vi "Dashboard Main.vi"() -> ()   [LabVIEW 2013]
uses:
  <vilib>/event_ctls.llb/eventvkey.ctl
  <vilib>/Rock Robotics/WPI/Dashboard/WPI_DashboardLogging Global.vi
  <vilib>/Utility/config.llb/Write Key (String).vi
  <vilib>/Utility/config.llb/Write Key (I32).vi
  <vilib>/Utility/config.llb/NI_LVConfig.lvlib
panel:
  out "Image Message":string="Timeout in Camera Communications"
  in  "Rec Mode":enum32{"Stop", "Record", "Playback"}(radio)
  in  "Dashboard Tab":T1(tab)
  out "Auto-Grab Trigger":bool
  out "Arm Resting":bool
  out "Arm Pos":dbl
  in  "Retract Speed":dbl=0.4
  out "Motor2":dbl
  out "Motor1":dbl
  out "Launch":bool
  out "Grab":bool
  out "Launch Speed":dbl
  out "Launcher V":dbl
  in  "Pass Speed":dbl=-0.4
  in  "Max Launch Speed":dbl=-1.0
  in  "Pass V":dbl=2.8
  in  "Truss Launch V":dbl=1.7
  in  "Max Launch V":dbl=2.8
  in  "Camera Settings":T2={"Frame Rate"=30, "Compression"=30, "Size"=1} {"Frame Rate" scale=1.0..30.0; "Size" items=["640x480", "320x240", "160x120"]}
  out "MotorSliders R":cluster{"MotorSlide1":dbl, "MotorSlide2":dbl} {"MotorSlide2" scale=-1.0..1.0 scale format="%#_2e"; "MotorSlide1" scale=-1.0..1.0 scale format="%#_2e"}
  out "MotorChart R":cluster{"Numeric":dbl, "Numeric":dbl}(graph)
  out "MotorSliders L":T3 {"MotorSlide4 2" scale=0.0..14.0 scale format="%#_2e"; "MotorSlide2" scale=-1.0..1.0 scale format="%#_2e"; "MotorSlide1" scale=-1.0..1.0 scale format="%#_2e"}
  out "MotorChart L":T4(graph)
  out "JS1 Z":dbl(slide) scale=-1.0..1.0 scale format="%#_2e"
  out "Joystick 1":cluster{"X":dbl, "Y":dbl}[](graph)
  out "JS Buttons 1":T5
  out "JS2 Z":dbl(slide) scale=-1.0..1.0 scale format="%#_2e"
  out "Joystick 2":cluster{"X":dbl, "Y":dbl}[](graph)
  out "JS Buttons 2":T5
  out "Mode":T6(ring)=enum."Auto Disabled"
  out "Camera IP":string
  out "fps":dbl format="%#.1g"
  out "Mbps":dbl format="%#.1g"
  in  "DB Camera Config":bool
  in  "Enable":bool
  out "Mbps 2":bool
  in  "Horizontal":bool
  in  "Third":dbl=2000.0
  in  "Second":dbl=2500.0
  in  "Forward1":dbl=-0.8
  in  "First":dbl=2000.0
  in  "wait3":dbl=0.8
  in  "wait2":dbl
  in  "wait1":dbl
  in  "wait":dbl
  in  "Forward":dbl=-0.8 step=0.1
  in  "Test Slider":dbl(slide) scale=0.0..100.0 scale format="%#_3g"
  in  "On/Off":bool caption="Solenoid"
  in  "Test Name":u16(ring) items=["Select the test to run...", "Example Test", "-------------------------------", "List of tests is built in robot code.", "Replace with your own automated tests."]
  in  "Test Tree":string(tree)
  in  "Motor":cluster{"Value":dbl, "Enable":bool} {"Value" scale=-1.0..1.0 scale format="%#_3g"}
  out "Progress":T7 {"Test Progress" scale=0.0..100.0}
  in  "Rev/Fwd":cluster{"Forward":bool, "Reverse":bool}
  in  "Test Ring":u16(ring) items=["Auto", "Fixed indoor", "Fixed outdoor 1", "Fixed outdoor 2", "Fixed fluorescent 1", "Fixed fluorescent 2", "Hold current"]
  in  "Listbox":i32(listbox)
  out "Tree":string(tree)
  out "Camera Image":T8(plugin-control)
  # "Left"
  # "Front"
  # "Right"
  # "Battery"
  # "Customize by placing controls and indicators here and name to\nmatch Dashboard Variables on robot."
  # "This tab is a great place for autonomous settings and validation.\nCustomize by placing controls and indicators here and name to\nmatch Dashboard Variables on robot."
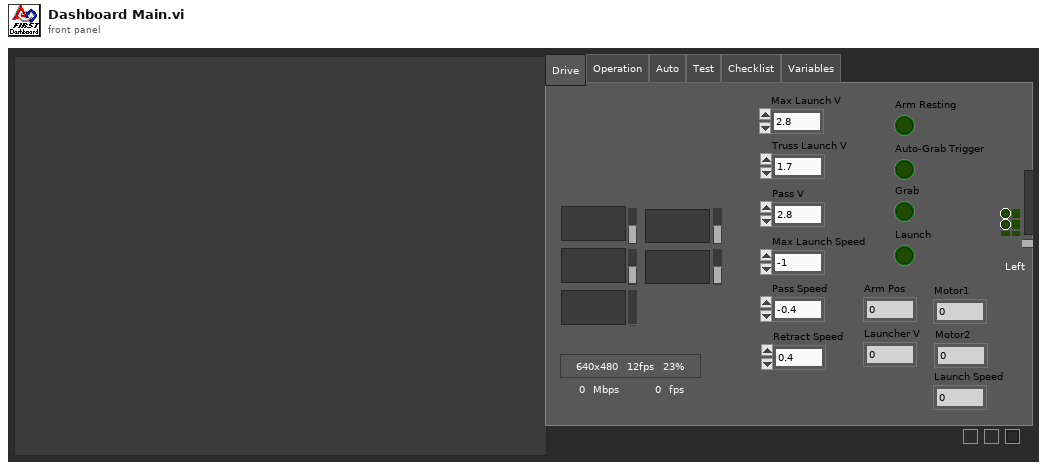
[diagram p1: front panel]
types:
  T1 = enum32{"Drive", "Operation", "Auto", "Test", "Checklist", "Variables"}
  T2 = cluster{"Frame Rate":i32, "Compression":i32, "Size":u16}
  T3 = cluster{"MotorSlide1":dbl, "MotorSlide2":dbl, "MotorSlide4 2":dbl}
  T4 = cluster{"Numeric":dbl, "Numeric":dbl, "Battery":sgl}
  T5 = cluster{bool, bool, bool, bool, bool, bool, bool, bool, bool, bool, bool, bool}
  T6 = enum8{"Tele-Op Disabled", "Tele-Op Enabled", "Auto Disabled", "Auto Enabled", "Test Disabled", "Test Enabled", ""}
  T7 = cluster{"Test Progress":u8, "Test Progress Text":string}
  T8 = typedef "IMAQ Image.ctl" = refnum<image>
  T9 = typedef "Image Type" = u32
  T10 = cluster{"Digital Inputs":bool[], "Digital Outputs":bool[]}
  T11 = cluster{"Competition mode":bool, "Robot Link":bool, "Autonomous":bool, "Enabled":bool, "E-Stop":bool, "Simulated":bool, "TestMode":bool, "Docked Window":bool}
  T12 = cluster{"wait":dbl, "wait1":dbl, "wait2":dbl, "wait3":dbl, "Forward":dbl, "Forward1":dbl, "First":dbl, "Second":dbl, "Third":dbl}
  T13 = cluster{"Boolean Array[0]":bool, "Boolean Array[1]":bool, "Boolean Array[2]":bool, "Boolean Array[3]":bool, "Boolean Array[4]":bool, "Boolean Array[5]":bool, "Boolean Array[6]":bool, "Boolean Array[7]":bool, "Boolean Array[8]":bool, "Boolean Array[9]":bool, "Boolean Array[10]":bool, "Boolean Array[11]":bool}
  T14 = typedef "NI_LVConfig.lvlib/Config Data RefNum.ctl" = refnum<k1>
  T15 = typedef "eventvkey.ctl" = enum16{"ASCII", "Enter", "Return", "Shift", "Ctrl", "Alt", "Cmd", "Opt", "Caps", "NumLock", "Clear", "Break", "Up", "Down", "Left", "Right", "Insert", "Delete", "Home", "End", "PageUp", "PageDown", "Escape", "Help", "Pause", "ScrollLock", "F1", "F2", "F3", "F4", "F5", "F6", "F7", "F8", "F9", "F10", "F11", "F12", "F13", "F14", "F15", "F16", "F17", "F18", "F19", "F20", "F21", "F22", "F23", "F24", "Play", "VolumeUp", "VolumeDown", "Mute", "Two Byte Char"}
  T16 = cluster{"Image Size":bool, "Image Type":bool, "Pixel Value":bool, "ROI Information":bool, "Zoom Factor":bool}
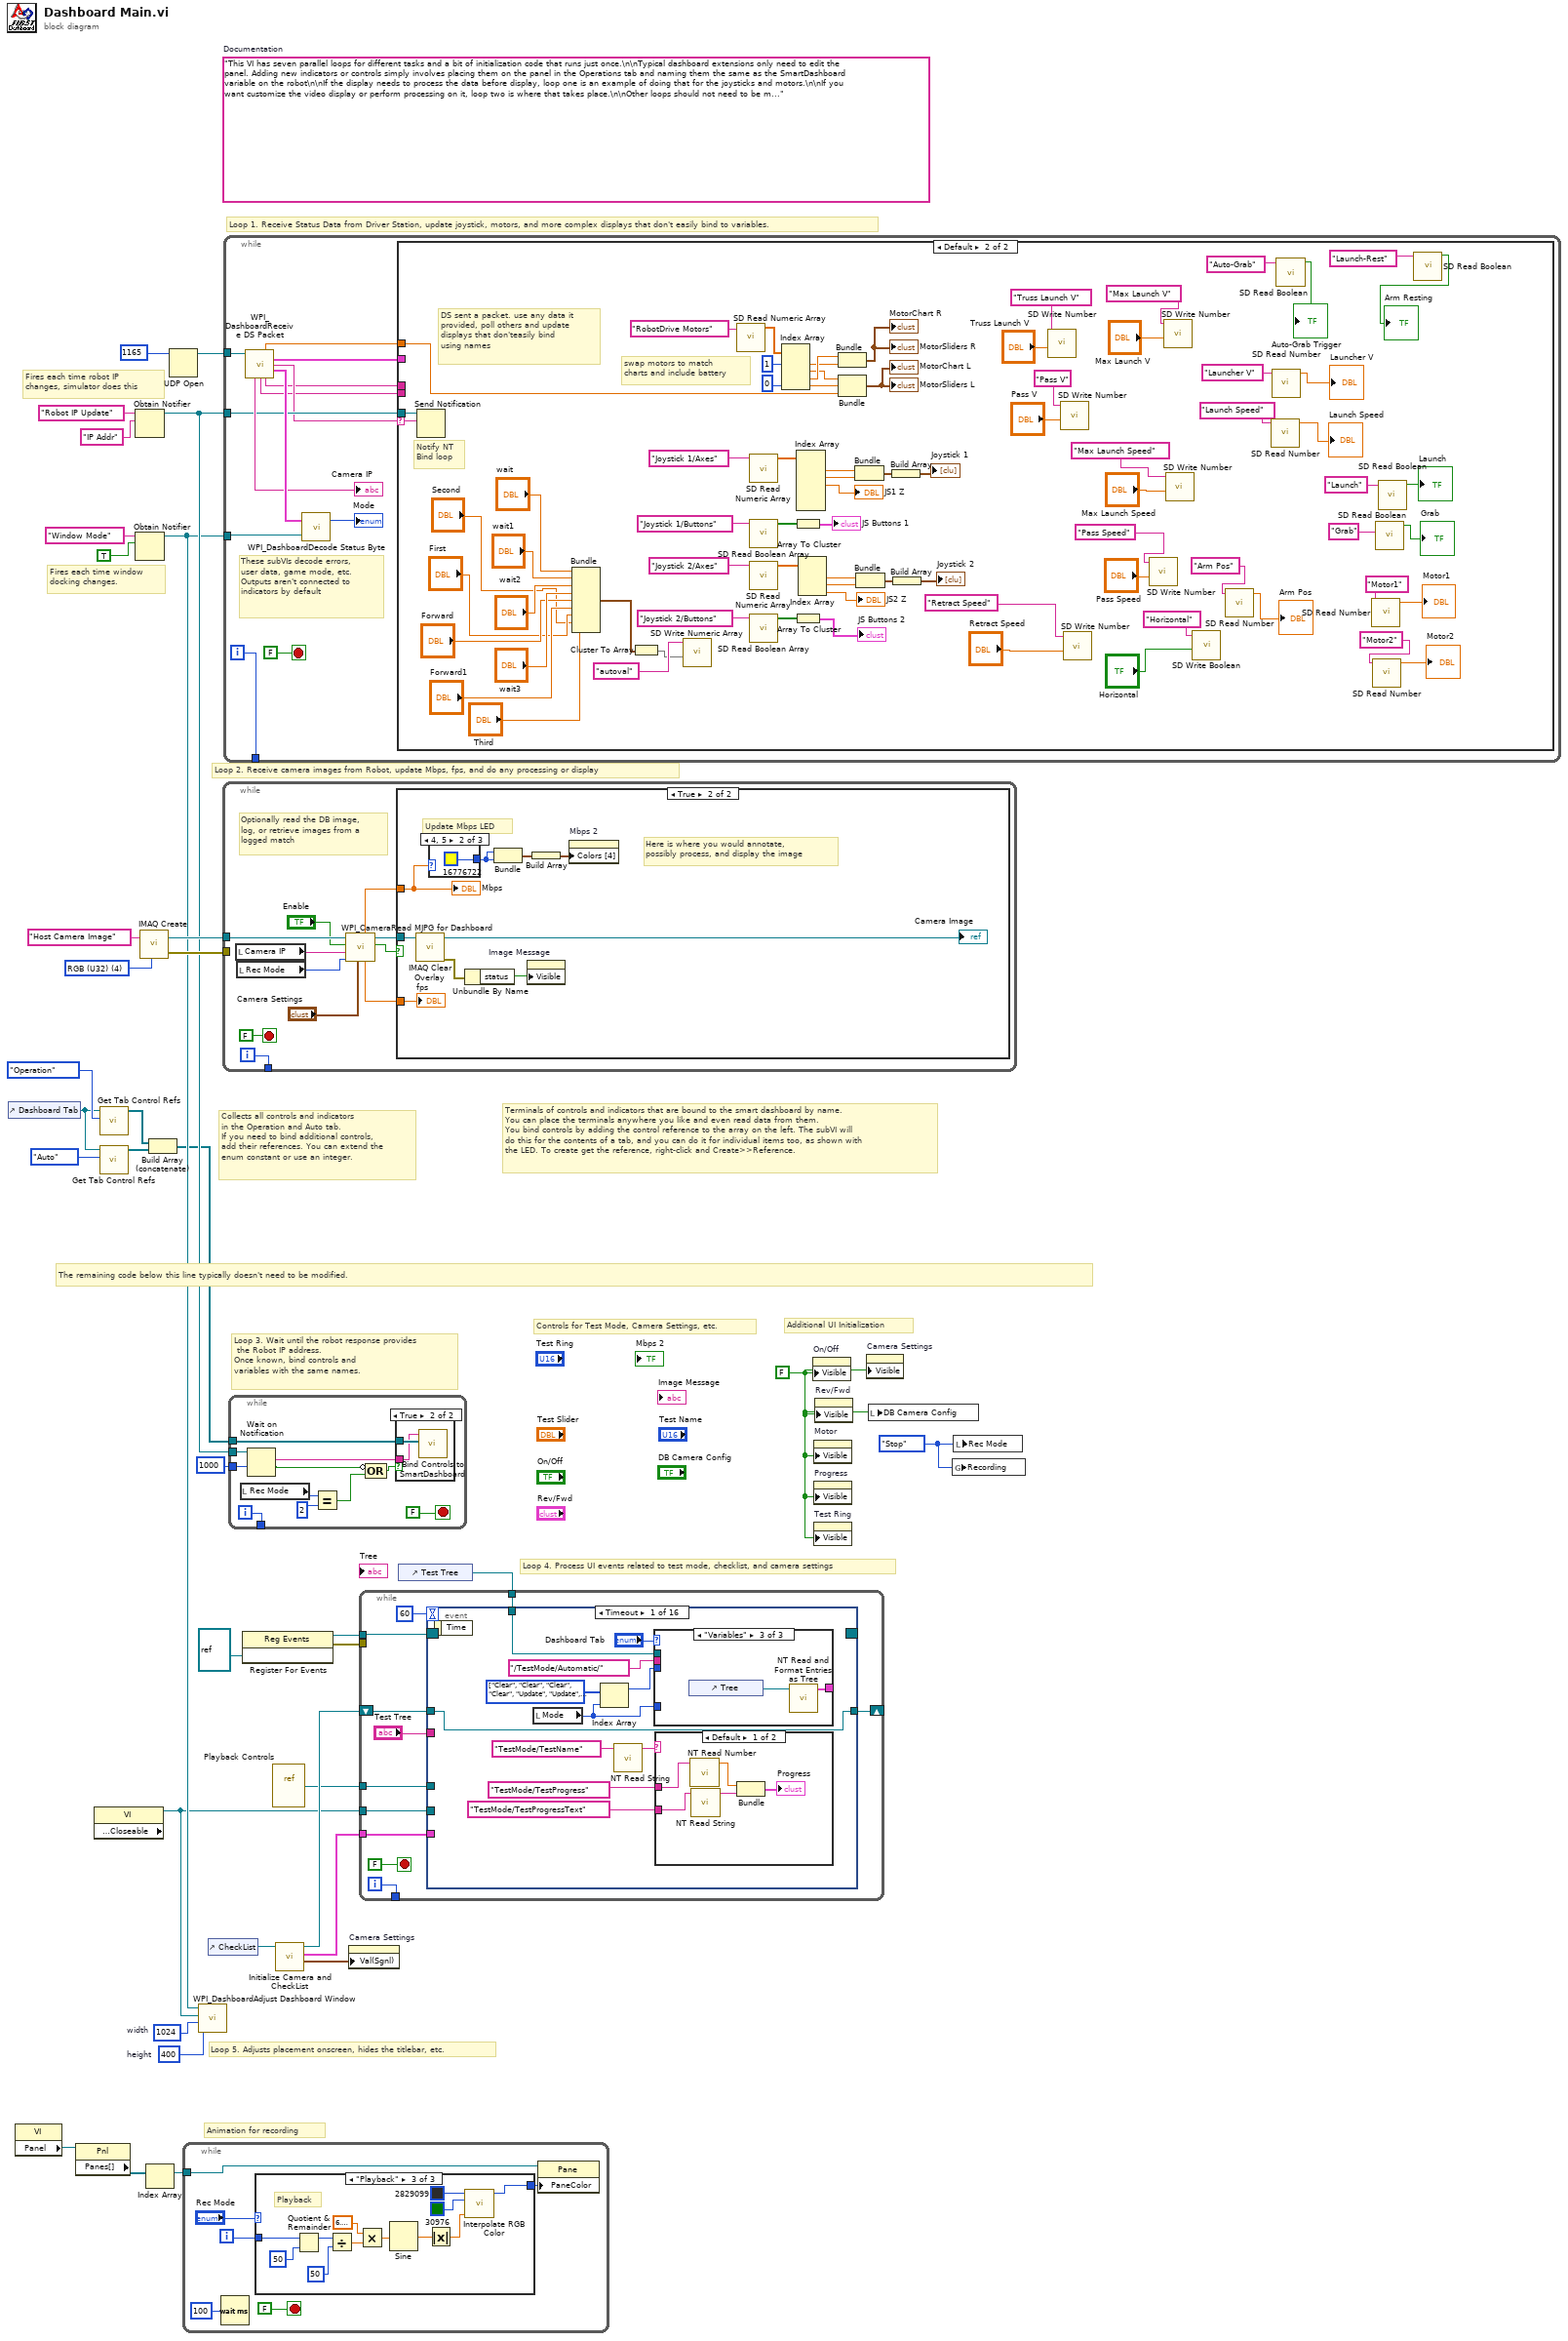
[diagram p0: block diagram]
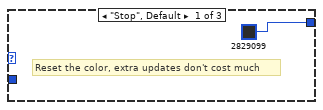
[diagram p2: hidden frame]
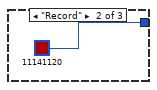
[diagram p3: hidden frame]
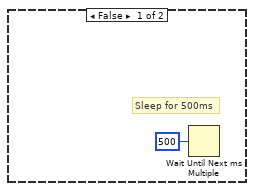
[diagram p5: hidden frame]
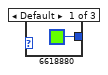
[diagram p6: hidden frame]
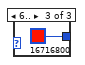
[diagram p7: hidden frame]
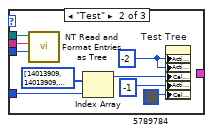
[diagram p9: hidden frame]
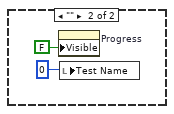
[diagram p10: hidden frame]
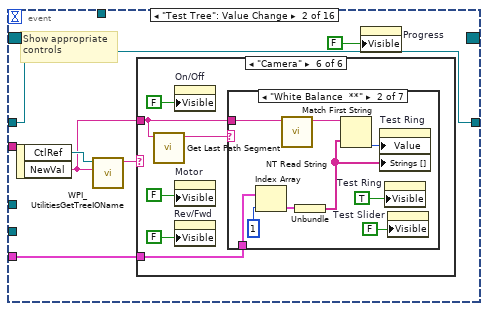
[diagram p11: hidden frame]
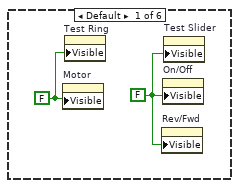
[diagram p12: hidden frame]
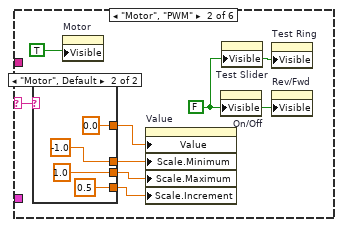
[diagram p13: hidden frame]
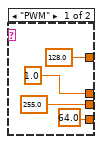
[diagram p14: hidden frame]
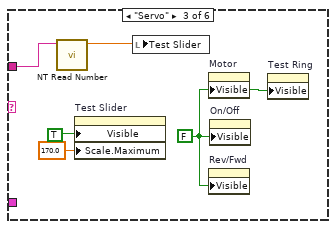
[diagram p15: hidden frame]
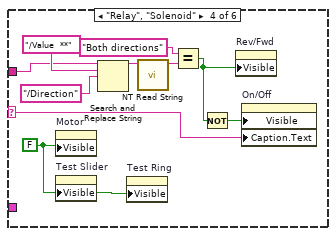
[diagram p16: hidden frame]
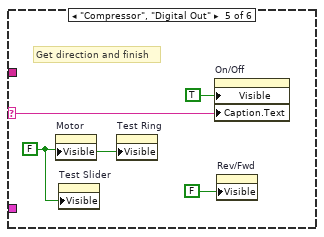
[diagram p17: hidden frame]
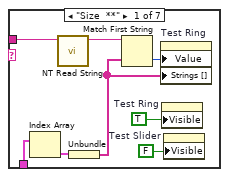
[diagram p18: hidden frame]
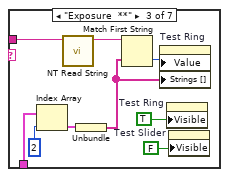
[diagram p19: hidden frame]
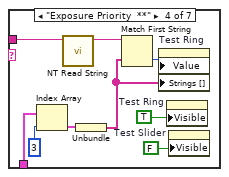
[diagram p20: hidden frame]
diagram:
  w7 = enum32{"Stop", "Record", "Playback"}."Stop" ("Rec Mode")
  w10 = 400  # height
  w11 = 1024  # width
  w24 = FALSE ("Visible")
  (unwired) "This VI has seven parallel loops for different tasks and a bit of initialization code that runs just once.\n\nTypical dashboard extensions only need to edit the panel. Adding new indicators or controls simply involves placing them on the panel in the Operations tab and naming them the same as the SmartDashboard variable on the robot\n\nIf the display needs to process the data before display, loop one is an example of doing that for the joysticks and motors.\n\nIf you want customize the video display or perform processing on it, loop two is where that takes place.\n\nOther loops should not need to be modified. They are pretty standard, and document the task they perform."  # Documentation
  w34 = T9 4 items=["Grayscale (U8)", "Grayscale (I16)", "Grayscale (SGL)", "Complex (CSG)", "RGB (U32)", "HSL (U32)", "RGB (U64)"] ("Image Type")
  # "Controls for Test Mode, Camera Settings, etc."
  # "Additional UI Initialization"
  # "Animation for recording"
  # "Fires each time robot IP\nchanges, simulator does this"
  # "Fires each time window\ndocking changes."
  # "Collects all controls and indicators\nin the Operation and Auto tab.\nIf you need to bind additional controls,\nadd their references. You can extend the\nenum constant or use an integer."
  # "The remaining code below this line typically doesn't need to be modified."
  # "Loop 4. Process UI events related to test mode, checklist, and camera settings"
  # "Terminals of controls and indicators that are bound to the smart dashboard by name.\nYou can place the terminals anywhere you like and even read data from them.\nYou bind controls by adding the control reference to the array on the left. The subVI will\ndo this for the contents of a tab, and you can do it for individual items too, as shown with\nthe LED. To create get the reference, right-click and Create>>Reference."
  # "Loop 3. Wait until the robot response provides\n the Robot IP address.\nOnce known, bind controls and\nvariables with the same names."
  # "Loop 5. Adjusts placement onscreen, hides the titlebar, etc."
  # "Loop 1. Receive Status Data from Driver Station, update joystick, motors, and more complex displays that don't easily bind to variables."
  # "Loop 2. Receive camera images from Robot, update Mbps, fps, and do any processing or display"
  n1 = control-ref of="Dashboard Tab"() -> (w5:refnum<vi>)
  n2 = property class="VI"() -> ("Panel"=w18:refnum<vi>)  [unwired: 2 in, 2 out]
  n3 = property class="Pnl"(reference=w18) -> ("Panes[]"=w19:refnum<vi>[])  [unwired: 1 in, 2 out]
  n4 = property class="VI" props=["Front Panel.Closeable"]() -> (reference out=w6:refnum<vi>)  [unwired: 2 in, 2 out]
  n5 = call <vilib>:"Get Tab Control Refs.vi"("Page Index"=T1."Operation" ("Dashboard Tab"), "TabControl in"=w5) -> ("ControlsOnPage"=w3:refnum<vi>[])  [unwired: 9 in]
  n6 = call <vilib>:"Get Tab Control Refs.vi"("Page Index"=T1."Auto" ("Dashboard Tab"), "TabControl in"=w5) -> ("ControlsOnPage"=w4:refnum<vi>[])  [unwired: 9 in]
  n7 = Obtain Notifier(name (unnamed)="Robot IP Update", notification data type="IP Addr" ("name (unnamed)")) -> (notifier out=w28:refnum<notifier>)  [unwired: 2 in, 2 out]
  n8 = Obtain Notifier(name (unnamed)="Window Mode", notification data type=TRUE) -> (notifier out=w9:refnum<notifier>)  [unwired: 2 in, 2 out]
  n9 = call "IMAQ Create"("Image Name"="Host Camera Image", "Image Type"=w34) -> ("New Image"=w32:T8, "error out"=w31:errorcluster)  [unwired: 2 in, 1 out]
  n10 = Index Array(array=w19) -> (element=w17:refnum<vi>)  [unwired: 1 in]
  n11 = Build Array (concatenate)(w3, w4) -> (w2:refnum<vi>[])
  n12 = UDP Open(11:u16 1165 ("port")) -> (port=w35:refnum<k16>)  [unwired: 2 in, 4 out]
  n13 = while {
    tunnel: w17 -> [w38]
    i -> [w41]
    stop <- FALSE stop-if-true
    n14 = Wait (ms)(milliseconds to wait=u32 100) -> ()  [unwired: 1 out]
    n15 = case shown="\"Playback\"" "Rec Mode" {
      tunnel: w41 -> [_ _ w56]
      tunnel: [u32 2829099 ("Base Color") u32 11141120 ("Target Color") w45] -> w37
      frame "Stop", Default {
        # "Reset the color, extra updates don't cost much"
      }
      frame "Record" {
      }
      frame "Playback" {
        # "Playback"
        n16 = Quotient & Remainder(x=w56, y=u32 50 ("milliseconds to wait")) -> (x-y*floor(x/y)=w52:u32)  [unwired: 1 out]
        n17 = Divide(x=w52, y=u32 50 ("milliseconds to wait")) -> (x/y=w49:dbl)
        n18 = Multiply(x=6.283185307179586, y=w49) -> (x*y=w54:dbl)
        n19 = Sine(x=w54) -> (sin(x)=w53:dbl)
        n20 = Absolute Value(x=w53) -> (abs(x)=w46:dbl)
        n21 = call "Interpolate RGB Color.vi"("Proportion"=w46, "Target Color"=u32 30976, "Base Color"=u32 2829099) -> ("Result Color"=w45:u32)  [unwired: 8 in]
      }
    }
    n22 = property class="Pane"(reference=w38, "PaneColor"=w37) -> ()  [unwired: 1 in, 2 out]
  }
  n23 = call <vilib>:"WPI_DashboardAdjust Dashboard Window.vi"("height"=w10, "width"=w11, "reference in"=w6, "Notifier in"=w9) -> ()  [unwired: 8 in]
  n24 = control-ref of="CheckList"() -> (w8:refnum<vi>)
  n25 = while {
    tunnel: w32 -> [w65]
    tunnel: w31 -> [_]
    tunnel: [w66] -> _
    i -> [w66]
    stop <- FALSE stop-if-true
    # "Optionally read the DB image,\nlog, or retrieve images from a\nlogged match"
    n26 = local read "Camera IP"() -> (w58:string)
    n27 = local read "Rec Mode"() -> (w57:enum32{"Stop", "Record", "Playback"})
    n28 = call <vilib>:"WPI_CameraRead MJPG for Dashboard.vi"("Camera Settings"="Camera Settings", "Rec Mode"=w57, "Camera IP"=w58, "Enable"="Enable", "Refnum in"=w65) -> ("Active"=w62:bool, "Refnum out"=w64:T8, "FPS"=w61:dbl, "Bandwidth (Mbps)"=w60:dbl)  [unwired: 3 in]
    n29 = case shown="True" w62 {
      tunnel: w64 -> [_ w72]
      tunnel: w60 -> [_ w71]
      tunnel: w61 -> [_ w69]
      frame False {
        # "Sleep for 500ms"
        n30 = Wait Until Next ms Multiple(millisecond multiple=u32 500) -> ()  [unwired: 1 out]
      }
      frame True {
        # "Here is where you would annotate,\npossibly process, and display the image"
        # "Update Mbps LED"
        n31 = call "IMAQ Clear Overlay"("Image"=w72) -> ("error out"=w76:errorcluster, "Image Out"=→"Camera Image":T8)  [unwired: 2 in, 7 out]
        n32 = case shown="4, 5" w71 {
          tunnel: [u32 6618880 ("Color Box") u32 16776722 ("Color Box") u32 16716800 ("Color Box")] -> w73
          frame Default {
          }
          frame 4, 5 {
          }
          frame 6.. {
          }
        }
        n33 = Unbundle By Name(w76) -> ("status"=w77:bool)
        n34 = Bundle("Color Box"=w73, "Color Box"=w73) -> (w75:cluster{"Color Box":u32, "Color Box":u32})  [unwired: 1 out]
        n35 = property on="Image Message" class="Str"("Visible"=w77) -> ()  [unwired: 2 in, 2 out]
        n36 = Build Array(w75) -> (w74:cluster{"Color Box":u32, "Color Box":u32}[])
        n37 = property on="Mbps 2" class="Bool (strict)"("Colors [4]"=w74) -> ()  [unwired: 2 in, 2 out]
        "Mbps" <- w71
        "fps" <- w69
      }
    }
  }
  n38 = while {
    tunnel: w35 -> [w91]
    tunnel: w28 -> [w86]
    tunnel: w9 -> [w90]
    tunnel: [w87] -> _
    i -> [w87]
    stop <- FALSE stop-if-true
    # "These subVIs decode errors, user data, game mode, etc.\nOutputs aren't connected to indicators by default"
    n39 = call <vilib>:"WPI_DashboardReceive DS Packet.vi"("Recv Socket"=w91) -> ("Battery"=w81:sgl, "Driver Station"=w82:T10, "Robot IP Address"=w85:string, "Status"=w92:T11, "Camera IP Address"=→"Camera IP":string, "Low Priority User Data"=w84:string, "High Priority User Data"=w83:string)  [unwired: 1 in, 7 out]
    n40 = call <vilib>:"WPI_DashboardDecode Status Byte.vi"("Window Mode Notifier"=w90, "Status"=w92) -> ("Mode"=→"Mode":T6)  [unwired: 1 out]
    n41 = case shown="Default" w85 {
      selector: w85 -> [_ w148]
      tunnel: w86 -> [_ w149]
      tunnel: w84 -> [_ _]
      tunnel: w83 -> [_ _]
      tunnel: w82 -> [_ _]
      tunnel: w81 -> [_ w147]
      frame "0.0.0.0" {
        # "DS not sending packets, or no robot exists yet.\nDon't poll the variables"
      }
      frame Default {
        # "Notify NT\nBind loop"
        # "DS sent a packet. use any data it\nprovided, poll others and update\ndisplays that don'teasily bind\nusing names"
        # "swap motors to match\ncharts and include battery"
        n42 = Send Notification(notification=w148, notifier=w149) -> ()  [unwired: 1 in, 2 out]
        n43 = Bundle("wait"="wait", "wait1"="wait1", "wait2"="wait2", "wait3"="wait3", "Forward"="Forward", "Forward1"="Forward1", "First"="First", "Second"="Second", "Third"="Third") -> (w103:T12)  [unwired: 1 in]
        n44 = Cluster To Array(cluster=w103) -> (array=w102:dbl[])
        n45 = call <vilib>:"SD Write Numeric Array.vi"("Numeric Array"=w102, "Name"="autoval") -> ()  [unwired: 8 in, 2 out]
        n46 = call <vilib>:"SD Read Numeric Array.vi"("Name"="RobotDrive Motors") -> ("Numeric Array"=w146:dbl[])  [unwired: 8 in, 2 out]
        n47 = call <vilib>:"SD Read Numeric Array.vi"("Name"="Joystick 1/Axes") -> ("Numeric Array"=w165:dbl[])  [unwired: 8 in, 2 out]
        n48 = call <vilib>:"SD Read Boolean Array.vi"("Name"="Joystick 1/Buttons") -> ("Boolean Array"=w167:bool[])  [unwired: 8 in, 2 out]
        n49 = call <vilib>:"SD Read Numeric Array.vi"("Name"="Joystick 2/Axes") -> ("Numeric Array"=w159:dbl[])  [unwired: 8 in, 2 out]
        n50 = call <vilib>:"SD Read Boolean Array.vi"("Name"="Joystick 2/Buttons") -> ("Boolean Array"=w158:bool[])  [unwired: 8 in, 2 out]
        n51 = Index Array(array=w146, index #1=1, index #4=0) -> (element #1=w142:dbl, element #2=w141:dbl, element #3=w143:dbl, element #4=w138:dbl)  [unwired: 2 in]
        n52 = Array To Cluster(array=w167) -> (cluster=→"JS Buttons 1":T13)
        n53 = Array To Cluster(array=w158) -> (cluster=→"JS Buttons 2":T13)
        n54 = Index Array(array=w165) -> (element #1=w162:dbl, element #2=w163:dbl, element #3=→"JS1 Z":dbl)  [unwired: 6 in, 3 out]
        n55 = Index Array(array=w159) -> (element #1=w154:dbl, element #2=w153:dbl, element #3=→"JS2 Z":dbl)  [unwired: 3 in]
        n56 = Bundle("Numeric"=w143, "Numeric"=w142) -> (→"MotorChart R" →"MotorSliders R":cluster{"Numeric":dbl, "Numeric":dbl})  [unwired: 1 in]
        n57 = Bundle("Numeric"=w141, "Numeric"=w138, "Battery"=w147) -> (→"MotorChart L" →"MotorSliders L":T4)  [unwired: 1 in]
        n58 = Bundle("Numeric"=w162, "Numeric"=w163) -> (w161:cluster{"Numeric":dbl, "Numeric":dbl})  [unwired: 1 in]
        n59 = Bundle("Numeric"=w154, "Numeric"=w153) -> (w155:cluster{"Numeric":dbl, "Numeric":dbl})  [unwired: 1 in]
        n60 = Build Array(w161) -> (→"Joystick 1":cluster{"Numeric":dbl, "Numeric":dbl}[])
        n61 = Build Array(w155) -> (→"Joystick 2":cluster{"Numeric":dbl, "Numeric":dbl}[])
        n62 = call <vilib>:"SD Write Number.vi"("Numeric"="Truss Launch V", "Name"="Truss Launch V") -> ()  [unwired: 8 in, 2 out]
        n63 = call <vilib>:"SD Write Number.vi"("Numeric"="Pass V", "Name"="Pass V") -> ()  [unwired: 8 in, 2 out]
        n64 = call <vilib>:"SD Write Number.vi"("Numeric"="Retract Speed", "Name"="Retract Speed") -> ()  [unwired: 8 in, 2 out]
        n65 = call <vilib>:"SD Write Number.vi"("Numeric"="Pass Speed", "Name"="Pass Speed") -> ()  [unwired: 8 in, 2 out]
        n66 = call <vilib>:"SD Write Number.vi"("Numeric"="Max Launch V", "Name"="Max Launch V") -> ()  [unwired: 8 in, 2 out]
        n67 = call <vilib>:"SD Write Number.vi"("Numeric"="Max Launch Speed", "Name"="Max Launch Speed") -> ()  [unwired: 8 in, 2 out]
        n68 = call <vilib>:"SD Write Boolean.vi"("Boolean"="Horizontal", "Name"="Horizontal") -> ()  [unwired: 8 in, 2 out]
        n69 = call <vilib>:"SD Read Number.vi"("Name"="Arm Pos") -> ("Numeric"=→"Arm Pos":dbl)  [unwired: 8 in, 2 out]
        n70 = call <vilib>:"SD Read Number.vi"("Name"="Launch Speed") -> ("Numeric"=→"Launch Speed":dbl)  [unwired: 8 in, 2 out]
        n71 = call <vilib>:"SD Read Number.vi"("Name"="Launcher V") -> ("Numeric"=→"Launcher V":dbl)  [unwired: 8 in, 2 out]
        n72 = call <vilib>:"SD Read Boolean.vi"("Name"="Auto-Grab") -> ("Boolean"=→"Auto-Grab Trigger":bool)  [unwired: 8 in, 2 out]
        n73 = call <vilib>:"SD Read Number.vi"("Name"="Motor1") -> ("Numeric"=→"Motor1":dbl)  [unwired: 8 in, 2 out]
        n74 = call <vilib>:"SD Read Number.vi"("Name"="Motor2") -> ("Numeric"=→"Motor2":dbl)  [unwired: 8 in, 2 out]
        n75 = call <vilib>:"SD Read Boolean.vi"("Name"="Grab") -> ("Boolean"=→"Grab":bool)  [unwired: 8 in, 2 out]
        n76 = call <vilib>:"SD Read Boolean.vi"("Name"="Launch") -> ("Boolean"=→"Launch":bool)  [unwired: 8 in, 2 out]
        n77 = call <vilib>:"SD Read Boolean.vi"("Name"="Launch-Rest") -> ("Boolean"=→"Arm Resting":bool)  [unwired: 8 in, 2 out]
      }
    }
  }
  n78 = while {
    tunnel: w2 -> [w181]
    tunnel: w28 -> [w179]
    tunnel: [w177] -> _
    tunnel: u32 1000 ("milliseconds to wait") -> [w176]
    i -> [w177]
    stop <- FALSE stop-if-true
    n79 = local read "Rec Mode"() -> (w172:enum32{"Stop", "Record", "Playback"})
    n80 = Wait on Notification(notifier=w179, timeout in ms (-1)=w176) -> (notification=w178:string, timed out?=w174:bool)  [unwired: 2 in, 2 out]
    n81 = Equal?(x=w172, y=u16 2 ("Rec Mode")) -> (x = y?=w173:bool)
    n82 = Compound Arithmetic op=OR(invert w174, w173) -> (w175:bool)
    n83 = case shown="True" w175 {
      tunnel: w181 -> [_ w183]
      tunnel: w178 -> [_ w182]
      frame False {
      }
      frame True {
        n84 = call <vilib>:"Bind Controls to SmartDashboard.vi"("Bound Control Refs"=w183, "Server IP Address"=w182) -> ()  [unwired: 10 in]
      }
    }
  }
  n85 = register-events(refnum<vi> refnum) -> (reference out=w15:refnum<event-registration>, error out=w14:errorcluster)  [unwired: 2 in]
  n86 = vi-ref "Playback Controls.vi"() -> (w16:refnum<vi>)
  n87 = call "Initialize Camera and CheckList.vi"("ListBox in"=w8) -> ("Cluster"=w22:cluster{"value":i32, "value":i32, "index":i32}, "Array"=w23:cluster{string[]}[], "File Refnum"=w21:T14)  [unwired: 8 in]
  n88 = property on="Camera Settings" class="Clust (strict)"("Val(Sgnl)"=w22) -> ()  [unwired: 2 in, 2 out]
  n89 = control-ref of="Test Tree"() -> (w20:refnum<vi>)
  n90 = while {
    tunnel: w23 -> [w191]
    shift-right: [w190] -> _
    shift-left: w21 -> [w189]
    tunnel: [w188] -> _
    tunnel: w20 -> [w187]
    tunnel: w16 -> [w186]
    tunnel: w15 -> [w185]
    tunnel: w14 -> [_]
    tunnel: w6 -> [w184]
    i -> [w188]
    stop <- FALSE stop-if-true
    n91 = event shown="[0] Timeout" {
      selector: w185 -> [_ _ _ _ _ _ _ _ _ _ _ _ _ _ _ _]
      dyn-events: [_ _ _ _ _ _ _ _ _ _ _ _ _ w429 _ _] -> _
      timeout: u32 60 ("milliseconds to wait") -> [_ _ _ _ _ _ _ _ _ _ _ _ _ _ _ _]
      tunnel: w187 -> [w201 _ _ _ _ _ _ _ _ _ _ _ _ _ _ _]
      tunnel: "Test Tree" -> [_ _ _ _ _ _ _ _ w398 w406 w408 w412 w420 _ _ _]
      tunnel: w191 -> [_ w225 _ _ _ _ w362 w392 _ _ _ _ _ _ _ _]
      tunnel: [w195 w224 w323 w328 w336 w348 w361 w385 w397 w404 w407 w411 w419 w431 w445 w446] -> w190
      tunnel: w189 -> [w195 w224 w323 w328 w336 w348 w360 w385 w397 w404 w407 w411 w419 w431 w445 w446]
      tunnel: w186 -> [_ _ _ _ _ _ _ _ _ _ _ _ _ w432 _ w449]
      tunnel: w184 -> [_ _ _ _ _ _ _ _ _ _ _ _ _ w427 _ _]
      event Timeout {
        w200 = enum16{"Update", "Clear"}[] [enum."Clear", enum."Clear", enum."Clear", enum."Clear", enum."Update", enum."Update", enum."Clear"] items=["Update", "Clear"]
        n92 = event-data() -> ()  [unwired: 1 in, 1 out]
        n93 = local read "Mode"() -> (w198:T6)
        n94 = Index Array(array=w200, index=w198) -> (element=w199:enum16{"Update", "Clear"})
        n95 = call <vilib>:"NT Read String.vi"("Name"="TestMode/TestName") -> ("String"=w204:string)  [unwired: 9 in, 1 out]
        n96 = case shown="\"Variables\"" "Dashboard Tab" {
          tunnel: w201 -> [_ w214 _]
          tunnel: "/TestMode/Automatic/" ("Name Pattern") -> [_ w213 _]
          tunnel: w199 -> [_ w212 _]
          tunnel: w198 -> [_ w210 _]
          tunnel: [_ _ w216] -> _
          frame "Operation", Default {
          }
          frame "Test" {
            w209 = -2 ("Active Item:Row Number")
            n97 = call <vilib>:"NT Read and Format Entries as Tree.vi"("Operation"=w212, "Name Pattern"=w213, "Tree Refnum"=w214) -> ()  [unwired: 7 in, 2 out]
            n98 = Index Array(array=u32[] [14013909, 14013909, 14013909, 14013909, 14013909, 16777215, 14013909], index=w210) -> (element=w208:u32)
            n99 = property on="Test Tree" class="Tree (strict)"("Active Item Row Number"=w209, "ActiveColNum"=w209, "CellBG"=w208, "Active Item Row Number"=-1 ("Active Item:Row Number"), "CellBG"=u32 5789784 ("Color Box")) -> ()  [unwired: 2 in, 2 out]
          }
          frame "Variables" {
            n100 = control-ref of="Tree"() -> (w215:refnum<vi>)
            n101 = call <vilib>:"NT Read and Format Entries as Tree.vi"("Tree Refnum"=w215) -> ("Formatted Strings"=w216:cluster{"Name":string, "Value":string}[])  [unwired: 9 in, 1 out]
          }
        }
        n102 = case shown="Default" w204 {
          tunnel: "TestMode/TestProgress" ("Name") -> [w218 _]
          tunnel: "TestMode/TestProgressText" ("Name") -> [w217 _]
          frame Default {
            n103 = call <vilib>:"NT Read Number.vi"("Name"=w218) -> ("Numeric"=w219:dbl)  [unwired: 9 in, 1 out]
            n104 = call <vilib>:"NT Read String.vi"("Name"=w217) -> ("String"=w220:string)  [unwired: 9 in, 1 out]
            n105 = Bundle("Numeric"=w219, "String"=w220) -> (→"Progress":cluster{"Numeric":dbl, "String":string})  [unwired: 1 in]
          }
          frame "" {
            n106 = property on="Progress" class="Clust (strict)"("Visible"=FALSE) -> ()  [unwired: 2 in, 2 out]
            n107 = local write "Test Name"(u16 0) -> ()
          }
        }
      }
      event "Test Tree": Value Change {
        # "Show appropriate\ncontrols"
        n108 = event-data() -> ("CtlRef"=w228:refnum<vi>, "NewVal"=w226:string)  [unwired: 1 in]
        n109 = call <vilib>:"WPI_UtilitiesGetTreeIOName.vi"("NewVal"=w226, "TreeControl in"=w228) -> ("I/O Name"=w229:string)  [unwired: 9 in]
        n110 = case shown="\"Camera\"" w229 {
          selector: w229 -> [_ w236 _ w254 w263 _]
          tunnel: w226 -> [_ _ w251 w253 _ w270]
          tunnel: w225 -> [_ _ _ _ _ w269]
          frame Default {
            w231 = FALSE ("Visible")
            w230 = FALSE ("Visible")
            n111 = property on="Motor" class="Clust (strict)"("Visible"=w230) -> ()  [unwired: 2 in, 2 out]
            n112 = property on="Test Ring" class="Ring (strict)"("Visible"=w230) -> ()  [unwired: 2 in, 2 out]
            n113 = property on="Rev/Fwd" class="Clust (strict)"("Visible"=w231) -> ()  [unwired: 2 in, 2 out]
            n114 = property on="On/Off" class="Bool (strict)"("Visible"=w231) -> ()  [unwired: 2 in, 2 out]
            n115 = property on="Test Slider" class="Slide (strict)"("Visible"=w231) -> ()  [unwired: 2 in, 2 out]
          }
          frame "Motor", "PWM" {
            w237 = FALSE ("Visible")
            n116 = case shown="\"Motor\", Default" w236 {
              tunnel: [1.0 ("Value") -1.0 ("Value")] -> w235
              tunnel: [255.0 ("Value") 1.0 ("Value")] -> w234
              tunnel: [128.0 ("Value") 0.0 ("Value")] -> w233
              tunnel: [64.0 ("Value") 0.5 ("Value")] -> w232
              frame "PWM" {
              }
              frame "Motor", Default {
              }
            }
            n117 = property on="Motor" class="Clust (strict)"("Visible"=TRUE) -> ()  [unwired: 2 in, 2 out]
            n118 = property on="Value" class="Slide (strict)"("Value"=w233, "Scale.Minimum"=w235, "Scale.Maximum"=w234, "Scale.Increment"=w232) -> ()  [unwired: 2 in, 2 out]
            n119 = property on="On/Off" class="Bool (strict)"("Visible"=w237) -> ()  [unwired: 2 in, 2 out]
            n120 = property on="Test Slider" class="Slide (strict)"("Visible"=w237) -> ()  [unwired: 2 in, 2 out]
            n121 = property on="Test Ring" class="Ring (strict)"("Visible"=w237) -> ()  [unwired: 2 in, 2 out]
            n122 = property on="Rev/Fwd" class="Clust (strict)"("Visible"=w237) -> ()  [unwired: 2 in, 2 out]
          }
          frame "Servo" {
            w249 = FALSE ("Visible")
            n123 = call <vilib>:"NT Read Number.vi"("Name"=w251) -> ("Numeric"=w250:dbl)  [unwired: 9 in, 1 out]
            n124 = property on="Test Slider" class="Slide (strict)"("Visible"=TRUE, "Scale.Maximum"=170.0 ("Scale.Range:Maximum")) -> ()  [unwired: 2 in, 2 out]
            n125 = local write "Test Slider"(w250) -> ()
            n126 = property on="Motor" class="Clust (strict)"("Visible"=w249) -> ()  [unwired: 2 in, 2 out]
            n127 = property on="Rev/Fwd" class="Clust (strict)"("Visible"=w249) -> ()  [unwired: 2 in, 2 out]
            n128 = property on="On/Off" class="Bool (strict)"("Visible"=w249) -> ()  [unwired: 2 in, 2 out]
            n129 = property on="Test Ring" class="Ring (strict)"("Visible"=w249) -> ()  [unwired: 2 in, 2 out]
          }
          frame "Relay", "Solenoid" {
            w252 = FALSE ("Visible")
            n130 = property on="Motor" class="Clust (strict)"("Visible"=w252) -> ()  [unwired: 2 in, 2 out]
            n131 = property on="Test Slider" class="Slide (strict)"("Visible"=w252) -> ()  [unwired: 2 in, 2 out]
            n132 = Search and Replace String(input string=w253, search string="/Value  **", replace string="/Direction") -> (result string=w259:string)  [unwired: 5 in, 3 out]
            n133 = property on="Test Ring" class="Ring (strict)"("Visible"=w252) -> ()  [unwired: 2 in, 2 out]
            n134 = call <vilib>:"NT Read String.vi"("Name"=w259) -> ("String"=w257:string)  [unwired: 9 in, 1 out]
            n135 = Equal?(x="Both directions", y=w257) -> (x = y?=w255:bool)
            n136 = Not(x=w255) -> (.not. x?=w256:bool)
            n137 = property on="Rev/Fwd" class="Clust (strict)"("Visible"=w255) -> ()  [unwired: 2 in, 2 out]
            n138 = property on="On/Off" class="Bool (strict)"("Visible"=w256, "Caption.Text"=w254) -> ()  [unwired: 2 in, 2 out]
          }
          frame "Compressor", "Digital Out" {
            w262 = FALSE ("Visible")
            # "Get direction and finish"
            n139 = property on="Motor" class="Clust (strict)"("Visible"=w262) -> ()  [unwired: 2 in, 2 out]
            n140 = property on="Test Slider" class="Slide (strict)"("Visible"=w262) -> ()  [unwired: 2 in, 2 out]
            n141 = property on="Test Ring" class="Ring (strict)"("Visible"=w262) -> ()  [unwired: 2 in, 2 out]
            n142 = property on="On/Off" class="Bool (strict)"("Visible"=TRUE, "Caption.Text"=w263) -> ()  [unwired: 2 in, 2 out]
            n143 = property on="Rev/Fwd" class="Clust (strict)"("Visible"=FALSE) -> ()  [unwired: 2 in, 2 out]
          }
          frame "Camera" {
            n144 = call <vilib>:"Get Last Path Segment.vi"("String in"=w270) -> ("String out"=w271:string)  [unwired: 10 in]
            n145 = property on="On/Off" class="Bool (strict)"("Visible"=FALSE) -> ()  [unwired: 2 in, 2 out]
            n146 = property on="Motor" class="Clust (strict)"("Visible"=FALSE) -> ()  [unwired: 2 in, 2 out]
            n147 = property on="Rev/Fwd" class="Clust (strict)"("Visible"=FALSE) -> ()  [unwired: 2 in, 2 out]
            n148 = case shown="\"White Balance  **\"" w271 {
              tunnel: w270 -> [w277 w286 w295 w304 w313 _ w319]
              tunnel: w269 -> [w275 w283 w292 w301 w310 _ _]
              frame "Size  **" {
                n149 = Index Array(array=w275) -> (element=w274:cluster{string[]})  [unwired: 1 in]
                n150 = call <vilib>:"NT Read String.vi"("Name"=w277) -> ("String"=w276:string)  [unwired: 9 in, 1 out]
                n151 = Unbundle(w274) -> (w272:string[])
                n152 = Match First String(2:w272, 3:w276) -> (0:w273:i32)  [unwired: 1 out]
                n153 = property on="Test Ring" class="Ring (strict)"("Value"=w273, "Strings []"=w272) -> ()  [unwired: 2 in, 2 out]
                n154 = property on="Test Ring" class="Ring (strict)"("Visible"=TRUE) -> ()  [unwired: 2 in, 2 out]
                n155 = property on="Test Slider" class="Slide (strict)"("Visible"=FALSE) -> ()  [unwired: 2 in, 2 out]
              }
              frame "White Balance  **" {
                n156 = Index Array(array=w283, index=1) -> (element=w284:cluster{string[]})
                n157 = call <vilib>:"NT Read String.vi"("Name"=w286) -> ("String"=w285:string)  [unwired: 9 in, 1 out]
                n158 = Unbundle(w284) -> (w281:string[])
                n159 = Match First String(2:w281, 3:w285) -> (0:w280:i32)  [unwired: 1 out]
                n160 = property on="Test Ring" class="Ring (strict)"("Value"=w280, "Strings []"=w281) -> ()  [unwired: 2 in, 2 out]
                n161 = property on="Test Ring" class="Ring (strict)"("Visible"=TRUE) -> ()  [unwired: 2 in, 2 out]
                n162 = property on="Test Slider" class="Slide (strict)"("Visible"=FALSE) -> ()  [unwired: 2 in, 2 out]
              }
              frame "Exposure  **" {
                n163 = Index Array(array=w292, index=2) -> (element=w293:cluster{string[]})
                n164 = call <vilib>:"NT Read String.vi"("Name"=w295) -> ("String"=w294:string)  [unwired: 9 in, 1 out]
                n165 = Unbundle(w293) -> (w289:string[])
                n166 = Match First String(2:w289, 3:w294) -> (0:w290:i32)  [unwired: 1 out]
                n167 = property on="Test Ring" class="Ring (strict)"("Value"=w290, "Strings []"=w289) -> ()  [unwired: 2 in, 2 out]
                n168 = property on="Test Ring" class="Ring (strict)"("Visible"=TRUE) -> ()  [unwired: 2 in, 2 out]
                n169 = property on="Test Slider" class="Slide (strict)"("Visible"=FALSE) -> ()  [unwired: 2 in, 2 out]
              }
              frame "Exposure Priority  **" {
                n170 = Index Array(array=w301, index=3) -> (element=w302:cluster{string[]})
                n171 = call <vilib>:"NT Read String.vi"("Name"=w304) -> ("String"=w303:string)  [unwired: 9 in, 1 out]
                n172 = Unbundle(w302) -> (w298:string[])
                n173 = Match First String(2:w298, 3:w303) -> (0:w299:i32)  [unwired: 1 out]
                n174 = property on="Test Ring" class="Ring (strict)"("Value"=w299, "Strings []"=w298) -> ()  [unwired: 2 in, 2 out]
                n175 = property on="Test Ring" class="Ring (strict)"("Visible"=TRUE) -> ()  [unwired: 2 in, 2 out]
                n176 = property on="Test Slider" class="Slide (strict)"("Visible"=FALSE) -> ()  [unwired: 2 in, 2 out]
              }
              frame "Color Enable  **" {
                n177 = Index Array(array=w310, index=4) -> (element=w311:cluster{string[]})
                n178 = call <vilib>:"NT Read String.vi"("Name"=w313) -> ("String"=w312:string)  [unwired: 9 in, 1 out]
                n179 = Unbundle(w311) -> (w307:string[])
                n180 = Match First String(2:w307, 3:w312) -> (0:w308:i32)  [unwired: 1 out]
                n181 = property on="Test Ring" class="Ring (strict)"("Value"=w308, "Strings []"=w307) -> ()  [unwired: 2 in, 2 out]
                n182 = property on="Test Ring" class="Ring (strict)"("Visible"=TRUE) -> ()  [unwired: 2 in, 2 out]
                n183 = property on="Test Slider" class="Slide (strict)"("Visible"=FALSE) -> ()  [unwired: 2 in, 2 out]
              }
              frame Default {
                n184 = property on="Test Ring" class="Ring (strict)"("Visible"=FALSE) -> ()  [unwired: 2 in, 2 out]
                n185 = property on="Test Slider" class="Slide (strict)"("Visible"=FALSE) -> ()  [unwired: 2 in, 2 out]
              }
              frame "Brightness  **", "Color Level  **", "Compression  **", "FPS  **", "Sharpness  **" {
                n186 = call <vilib>:"NT Read Number.vi"("Name"=w319) -> ("Numeric"=w318:dbl)  [unwired: 9 in, 1 out]
                n187 = local write "Test Slider"(w318) -> ()
                n188 = property on="Test Slider" class="Slide (strict)"("Visible"=TRUE, "Scale.Maximum"=100.0 ("Scale.Range:Maximum")) -> ()  [unwired: 2 in, 2 out]
                n189 = property on="Test Ring" class="Ring (strict)"("Visible"=FALSE) -> ()  [unwired: 2 in, 2 out]
              }
            }
          }
        }
        n190 = property on="Progress" class="Clust (strict)"("Visible"=FALSE) -> ()  [unwired: 2 in, 2 out]
      }
      event "Test Name": Mouse Enter {
        # "Populate the ring with the list of tests"
        n191 = event-data() -> ()  [unwired: 1 in, 1 out]
        n192 = call <vilib>:"NT Read String Array.vi"("Name"="TestMode/TestList") -> ("String Array"=w327:string[])  [unwired: 9 in, 1 out]
        n193 = Build Array (concatenate)("Select the test to run...", w327) -> (w326:string[])
        n194 = property on="Test Name" class="Ring (strict)"("Strings []"=w326) -> ()  [unwired: 2 in, 2 out]
      }
      event "Test Name": Value Change {
        w329 = FALSE ("Visible")
        # "Tell the robot the test name to run"
        n195 = event-data() -> ("NewVal"=w333:u16)  [unwired: 1 in]
        n196 = property on="Test Name" class="Ring (strict)"() -> ("Strings []"=w334:string[])  [unwired: 2 in, 2 out]
        n197 = local write "Progress"(T7 {"Test Progress"=0, "Test Progress Text"=""} ("Progress")) -> ()
        n198 = Index Array(array=w334, index=w333) -> (element=w332:string)
        n199 = call <vilib>:"NT Write String.vi"("String"=w332, "Name"="TestMode/TestName") -> ()  [unwired: 9 in, 1 out]
        n200 = property on="Progress" class="Clust (strict)"("Visible"=TRUE) -> ()  [unwired: 2 in, 2 out]
        n201 = property on="Motor" class="Clust (strict)"("Visible"=w329) -> ()  [unwired: 2 in, 2 out]
        n202 = property on="Test Slider" class="Slide (strict)"("Visible"=w329) -> ()  [unwired: 2 in, 2 out]
        n203 = property on="On/Off" class="Bool (strict)"("Visible"=w329) -> ()  [unwired: 2 in, 2 out]
        n204 = property on="Rev/Fwd" class="Clust (strict)"("Visible"=w329) -> ()  [unwired: 2 in, 2 out]
        n205 = property on="Test Ring" class="Ring (strict)"("Visible"=w329) -> ()  [unwired: 2 in, 2 out]
      }
      event "Listbox": Double Click {
        n206 = event-data() -> ("PlatMods.Shift"=w337:bool, "Row"=w339:i32)  [unwired: 1 in]
        n207 = case shown="True" w337 {
          tunnel: w339 -> [w343 _]
          tunnel: 1 -> [w342 _]
          frame False {
            n208 = property on="Listbox" class="LstBox (strict)"() -> ("Item Symbols"=w341:i32[])  [unwired: 2 in, 2 out]
            n209 = Replace Array Subset(array=w341, new element=w342, index=w343) -> (w340:i32[])
            n210 = property on="Listbox" class="LstBox (strict)"("Item Symbols"=w340) -> ()  [unwired: 2 in, 2 out]
          }
          frame True {
            w344 = 0 ("Top Row")
            n211 = property on="Listbox" class="LstBox (strict)"() -> ("Number of Rows"=w346:u32)  [unwired: 2 in, 2 out]
            n212 = Initialize Array(0, w346) -> (w345:i32[])
            n213 = property on="Listbox" class="LstBox (strict)"("Top Row"=w344, "Value"=w344, "Item Symbols"=w345) -> ()  [unwired: 2 in, 2 out]
          }
        }
      }
      event "Listbox": Key Down {
        n214 = event-data() -> ("VKey"=w350:T15)  [unwired: 1 in]
        n215 = case shown="\"Left\", \"Right\"" w350 {
          selector: w350 -> [w355 _]
          tunnel: eventvkey."Left" ("VKey") -> [w353 _]
          frame "Left", "Right" {
            n216 = Equal?(x=w353, y=w355) -> (x = y?=w354:bool)
            n217 = Select(t=0, s=w354, f=1) -> (s? t:f=w356:i32)
            n218 = property on="Listbox" class="LstBox (strict)"() -> ("Item Symbols"=w359:i32[])  [unwired: 2 in, 2 out]
            n219 = Replace Array Subset(array=w359, new element=w356, index="Listbox") -> (w358:i32[])
            n220 = property on="Listbox" class="LstBox (strict)"("Item Symbols"=w358) -> ()  [unwired: 2 in, 2 out]
          }
          frame Default {
          }
        }
      }
      event "DB Camera Config": Value Change {
        n221 = event-data() -> ("NewVal"=w363:bool)  [unwired: 1 in]
        n222 = case shown="False" w363 {
          tunnel: w362 -> [w372 _]
          tunnel: [w365 w383] -> w361
          tunnel: w360 -> [w364 w383]
          frame False {
            w379 = "Camera"
            w382 = FALSE ("Visible")
            n223 = local read "Camera Settings"() -> (w371:T2)
            n224 = Index Array(array=w372) -> (element=w375:cluster{string[]})  [unwired: 1 in]
            n225 = Unbundle(w371) -> ("Frame Rate"=w370:i32, "Compression"=w369:i32, "Size"=w373:u16)
            n226 = Unbundle(w375) -> (w374:string[])
            n227 = Index Array(array=w374, index=w373) -> (element=w368:string)
            n228 = call-poly <vilib>:"Write Key.vi"("section"=w379, "value"=w368, "key"="Size", "refnum"=w364) -> ("refnum out"=w381:T14)  [unwired: 2 in, 5 out]
            n229 = call-poly <vilib>:"Write Key.vi"("section"=w379, "value"=w370, "key"="FrameRate", "refnum"=w381) -> ("refnum out"=w380:T14)  [unwired: 1 in, 6 out]
            n230 = property on="Camera Settings" class="Clust (strict)"("Visible"=w382) -> ()  [unwired: 2 in, 2 out]
            n231 = local write "DB Camera Config"(w382) -> ()
            n232 = call-poly <vilib>:"Write Key.vi"("section"=w379, "value"=w369, "key"="Compression", "refnum"=w380) -> ("refnum out"=w366:T14)  [unwired: 1 in, 6 out]
            n233 = call <vilib>:"Close Config Data.vi"("refnum"=w366) -> ("file path"=w367:path)  [unwired: 2 in, 8 out]
            n234 = call <vilib>:"Open Config Data.vi"("configuration file path"=w367) -> ("refnum"=w365:T14)  [unwired: 8 in, 2 out]
          }
          frame True {
            n235 = property on="Camera Settings" class="Clust (strict)"("Visible"=TRUE) -> ()  [unwired: 2 in, 2 out]
          }
        }
      }
      event "Camera Settings": Value Change {
        n236 = event-data() -> ("NewVal"=w396:T2)  [unwired: 1 in]
        n237 = Index Array(array=w392) -> (element=w391:cluster{string[]})  [unwired: 1 in]
        n238 = Unbundle(w396) -> ("Frame Rate"=w387:i32, "Compression"=w386:i32, "Size"=w389:u16)
        n239 = Unbundle(w391) -> (w390:string[])
        n240 = Index Array(array=w390, index=w389) -> (element=w388:string)
        n241 = Format Into String(format string="%s   %dfps   %d%%", w388, w387, w386) -> (resulting string=w393:string)  [unwired: 2 in, 1 out]
        n242 = Build Array(w393) -> (w394:string[])
        n243 = property on="DB Camera Config" class="Bool (strict)"("Strings [4]"=w394) -> ()  [unwired: 2 in, 2 out]
      }
      event "Motor.Enable": Value Change {
        n244 = event-data() -> ("NewVal"=w402:bool)  [unwired: 1 in]
        n245 = Unbundle("Motor") -> ("Value"=w401:dbl)  [unwired: 1 out]
        n246 = Select(t=w401, s=w402, f=0.0) -> (s? t:f=w399:dbl)
        n247 = call <vilib>:"NT Write Number.vi"("Numeric"=w399, "Name"=w398) -> ()  [unwired: 9 in, 1 out]
      }
      event "Test Slider": Value Change {
        n248 = event-data() -> ("NewVal"=w405:dbl)  [unwired: 1 in]
        n249 = call <vilib>:"NT Write Number.vi"("Numeric"=w405, "Name"=w406) -> ()  [unwired: 9 in, 1 out]
      }
      event "On/Off": Value Change {
        n250 = event-data() -> ("NewVal"=w410:bool)  [unwired: 1 in]
        n251 = Boolean To (0,1)(Boolean=w410) -> (0, 1=w409:i16)
        n252 = call <vilib>:"NT Write Number.vi"("Numeric"=w409, "Name"=w408) -> ()  [unwired: 9 in, 1 out]
      }
      event "Rev/Fwd": Value Change {
        n253 = event-data() -> ("NewVal.Forward"=w418:bool, "NewVal.Reverse"=w417:bool)  [unwired: 1 in]
        n254 = Boolean To (0,1)(Boolean=w418) -> (0, 1=w414:i16)
        n255 = Boolean To (0,1)(Boolean=w417) -> (0, 1=w416:i16)
        n256 = Negate(x=w416) -> (-x=w415:i16)
        n257 = Add(x=w414, y=w415) -> (x+y=w413:i16)
        n258 = call <vilib>:"NT Write Number.vi"("Numeric"=w413, "Name"=w412) -> ()  [unwired: 9 in, 1 out]
      }
      event "Test Ring": Value Change {
        n259 = event-data() -> ("NewVal"=w422:u16)  [unwired: 1 in]
        n260 = property on="Test Ring" class="Ring (strict)"() -> ("Strings []"=w423:string[])  [unwired: 2 in, 2 out]
        n261 = Index Array(array=w423, index=w422) -> (element=w421:string)
        n262 = call <vilib>:"NT Write String.vi"("String"=w421, "Name"=w420) -> ()  [unwired: 9 in, 1 out]
      }
      event "Rec Mode": Value Change {
        # "Update globals for recording mode and path to read log from.\nClear when logging and let NetworkTables set path for vision to\nuse."
        n263 = event-data() -> ("NewVal"=w433:enum32{"Stop", "Record", "Playback"})  [unwired: 1 in]
        n264 = global write "WPI_DashboardLogging Global.vi" "Logging Filename"(path "") -> ()
        n265 = case shown="\"Stop\", \"Record\"" w433 {
          tunnel: w432 -> [_ w435 w443]
          tunnel: [_ _ w442] -> w429
          tunnel: [_ _ w441] -> _
          tunnel: w427 -> [_ _ w439]
          tunnel: cluster{i32, i32} {-250, 170} -> [_ _ w438]
          tunnel: [_ _ T16 {"Image Size"=TRUE, "Image Type"=TRUE, "Pixel Value"=TRUE, "ROI Information"=TRUE, "Zoom Factor"=FALSE} ("Image Information Shown:All Elements")] -> w425
          tunnel: [_ _ TRUE ("Zoom Factor")] -> w424
          frame Default {
          }
          frame "Stop", "Record" {
            # "Place Window too"
            n266 = invoke class="VI" method="FP.Close"(reference=w435) -> (reference out=w434:refnum<vi>)  [unwired: 2 in, 2 out]
            n267 = invoke class="VI" method="Abort VI"(reference=w434) -> ()  [unwired: 2 in, 3 out]
          }
          frame "Playback" {
            n268 = call "Open Playback Panel.vi"("Offset"=w438, "DB VI Ref"=w439, "Playback in"=w443) -> ("Playback out"=w440:refnum<vi>)  [unwired: 8 in]
            n269 = register-events(w440) -> (reference out=w442:refnum<event-registration>, error out=w441:errorcluster)  [unwired: 2 in]
          }
        }
        n270 = global write "WPI_DashboardLogging Global.vi" "Recording"(w433) -> ()
        n271 = property on="Camera Image" class="ImageControl"("Image Information Shown"=w425, "Image Information Visible"=w424) -> ()  [unwired: 2 in, 2 out]
        n272 = call <vilib>:"WPI_DashboardNT Log FieldName Cache.vi"("Operation"=enum16{"Lookup/Add", "Index", "Clear"}."Clear") -> ()  [unwired: 8 in, 3 out]
      }
      event Panel Close {
        w444 = enum32{"Stop", "Record", "Playback"}."Stop" ("Rec Mode")
        n273 = event-data() -> ()  [unwired: 1 in, 4 out]
        n274 = local write "Rec Mode"(w444) -> ()
        n275 = global write "WPI_DashboardLogging Global.vi" "Recording"(w444) -> ()
      }
      event Panel Close {
        # "Abort playback window and ourself"
        n276 = event-data() -> ()  [unwired: 1 in, 4 out]
        n277 = invoke class="VI" method="FP.Close"(reference=w449) -> (reference out=w448:refnum<vi>)  [unwired: 2 in, 2 out]
        n278 = invoke class="VI" method="Abort VI"(reference=w448) -> (error out=w447:errorcluster)  [unwired: 2 in, 2 out]
        n279 = invoke class="VI" method="Abort VI"(error in=w447) -> ()  [unwired: 2 in, 3 out]
      }
    }
  }
  n280 = property on="On/Off" class="Bool (strict)"("Visible"=w24) -> ()  [unwired: 2 in, 2 out]
  n281 = property on="Motor" class="Clust (strict)"("Visible"=w24) -> ()  [unwired: 2 in, 2 out]
  n282 = property on="Progress" class="Clust (strict)"("Visible"=w24) -> ()  [unwired: 2 in, 2 out]
  n283 = property on="Test Ring" class="Ring (strict)"("Visible"=w24) -> ()  [unwired: 2 in, 2 out]
  n284 = property on="Rev/Fwd" class="Clust (strict)"("Visible"=w24) -> ()  [unwired: 2 in, 2 out]
  n285 = property on="Camera Settings" class="Clust (strict)"("Visible"=w24) -> ()  [unwired: 2 in, 2 out]
  n286 = local write "DB Camera Config"(w24) -> ()
  n287 = global write "WPI_DashboardLogging Global.vi" "Recording"(w7) -> ()
  n288 = local write "Rec Mode"(w7) -> ()
